vi "DSF.Engine.Memory.Buffer.Get Buffer Config.vi"(8 "error in (no error)":errorcluster, 11 "Buffer in":refnum<class "DSF.Engine.Memory.Buffer.lvclass">) -> (0 "error out":errorcluster, 2 "Buffer Config":refnum<class "DSF.Memory.Buffer.Config.lvclass">, 3 "Buffer out":refnum<class "DSF.Engine.Memory.Buffer.lvclass">)   [LabVIEW 2016, in "DSF.Engine.lvlib" / "DSF.Engine.Memory.Buffer.lvclass"]
uses:
  DSF.Engine.Memory.Buffer.lvclass
  DSF.Memory.Buffer.Config.lvclass
  DSF.Engine.Memory.Buffer.lvclass/DSF.Engine.Memory.Buffer.ctl
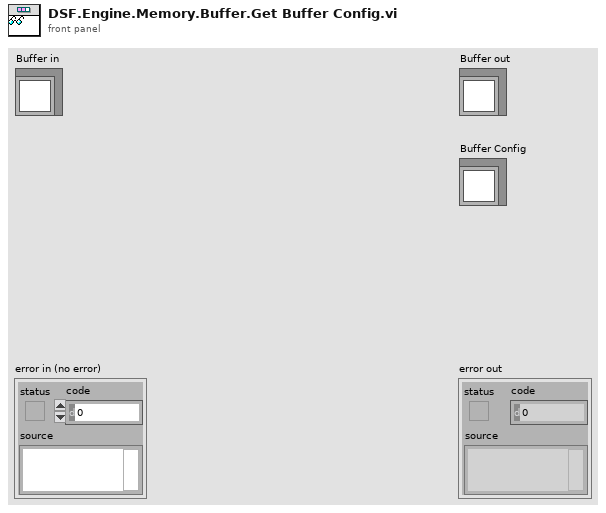
[diagram p1: front panel]
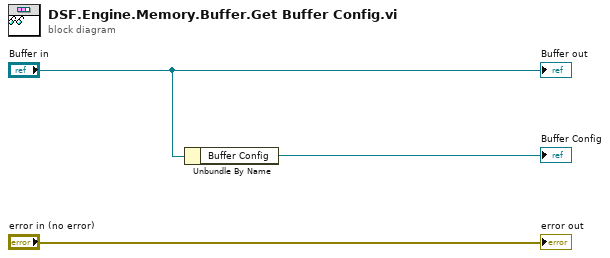
[diagram p0: block diagram]
diagram:
  n1 = Unbundle By Name("Buffer in") -> ("Buffer Config"=→"Buffer Config":refnum<class "DSF.Memory.Buffer.Config.lvclass">)
  "error out" <- "error in (no error)"
  "Buffer out" <- "Buffer in"
